vi "PhidgetGetChannelName.vi"(8 "error in":errorcluster, 11 "Device In":u64) -> (0 "error out":errorcluster, 2 "ChannelName":string, 3 "Device Out":u64)   [LabVIEW 2012, in "Phidget Common.lvlib"]
doc: "${ChannelName:Header}"
uses:
  <instrlib>/Phidgets/Phidget Common/Phidget Common.lvlib
  <vilib>/Utility/importsl/GetValueByPointer/datatype.ctl
  <vilib>/Utility/importsl/GetValueByPointer/GetValueByPointer.xnode
  phidget22.dll
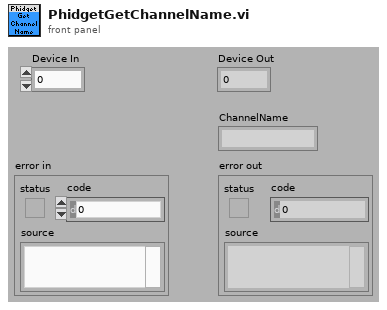
[diagram p1: front panel]
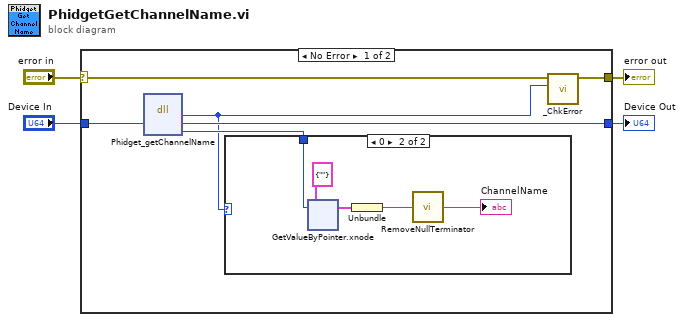
[diagram p0: block diagram]
diagram:
  n1 = case shown="No Error" "error in" {
    selector: "error in" -> [w9 w31]
    tunnel: [w8 w31] -> w3
    tunnel: [w7 w30] -> w2
    tunnel: "Device In" -> [w10 w30]
    frame No Error {
      n2 = dll-call lib="phidget22.*" fn="Phidget_getChannelName"("phid"=w10) -> ("return type"=w5:i32, "phid"=w7:u64, "DeviceLabel"=w6:u64)  [unwired: 4 in, 2 out]
      n3 = case shown="0" w5 {
        tunnel: w6 -> [_ w15]
        frame -1, Default {
        }
        frame 0 {
          n4 = xnode "GetValueByPointer.xnode"("Pointer"=w15, "InputType"=cluster{string} {""}) -> ("Output"=w13:cluster{string})  [unwired: 2 in, 1 out]
          n5 = Unbundle(w13) -> (w12:string)
          n6 = call <instrlib>:"RemoveNullTerminator.vi"("inString"=w12) -> ("outString"=→"ChannelName":string)
        }
      }
      n7 = call <instrlib>:"_ChkError.vi"("Return Code"=w5, "error in (no error)"=w9) -> ("error out"=w8:errorcluster)  [unwired: 9 in]
    }
    frame Error {
    }
  }
  "error out" <- w3
  "Device Out" <- w2
